vi "DllFxpSubTemp.vi"(6 "ready for output":bool, 9 "input valid":bool, 10 "y":fxp<+/-,16,1>, 11 "x":fxp<+/-,16,1>) -> (1 "output valid":bool, 2 "overflow?":bool, 3 "z":fxp<+/-,17,2> format="%.16g", 4 "ready for input":bool)   [LabVIEW 2017]
uses:
  <vilib>/rvi/FXPMathLib/FxpSub/subVIs/nifxpmath_Sub_SimConfig.ctl
  <vilib>/fxp/LVFixedPointQuantizationPolicyTypeDef.ctl
  <vilib>/fxp/LVFixedPointOverflowPolicyTypeDef.ctl
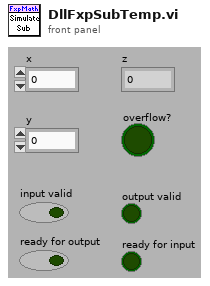
[diagram p1: front panel]
types:
  T1 = typedef "nifxpmath_Sub_SimConfig.ctl" = cluster{"kXSigned":bool, "kXWl":u32, "kXIwl":i32, "kYSigned":bool, "kYWl":u32, "kYIwl":i32, "kZSigned":bool, "kZWl":u32, "kZIwl":i32, "Fixed-Point:Quantization Policy":T2, "Fixed-Point:Overflow Policy":T3, "OutputRegister":bool, "SupportSCTL?":bool}
  T2 = typedef "LVFixedPointQuantizationPolicyTypeDef.ctl" = enum32{"Truncate", "Round-Half-Up (Asymmetric)", "Round-Half-Even"}
  T3 = typedef "LVFixedPointOverflowPolicyTypeDef.ctl" = enum32{"Wrap", "Saturate"}
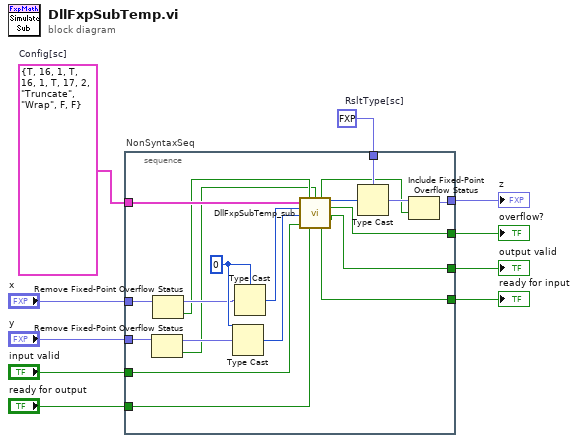
[diagram p0: block diagram]
diagram:
  w1 = T1 {"kXSigned"=TRUE, "kXWl"=16, "kXIwl"=1, "kYSigned"=TRUE, "kYWl"=16, "kYIwl"=1, "kZSigned"=TRUE, "kZWl"=17, "kZIwl"=2, "Fixed-Point:Quantization Policy"=enum."Truncate", "Fixed-Point:Overflow Policy"=enum."Wrap", "OutputRegister"=FALSE, "SupportSCTL?"=FALSE}  # Config[sc]
  w6 = fxp<+,17,2> 0.0  # RsltType[sc]
  n1 = stacked-sequence "NonSyntaxSeq" {
    tunnel: "x" -> [w19]
    tunnel: "y" -> [w16]
    tunnel: w6 -> [w30]
    tunnel: [w11] -> w5
    tunnel: "input valid" -> [w26]
    tunnel: [w24] -> w4
    tunnel: [w21] -> w2
    tunnel: [w20] -> w3
    tunnel: "ready for output" -> [w23]
    tunnel: w1 -> [w22]
    frame #0 {
      w29 = u64 0
      n2 = Remove Fixed-Point Overflow Status(3:w16) -> (0:w14:bool, 1:w15:fxp<+/-,16,1>)
      n3 = Remove Fixed-Point Overflow Status(3:w19) -> (0:w17:bool, 1:w18:fxp<+/-,16,1>)
      n4 = Type Cast(type=w29, x=w15) -> (*(type *) &x=w27:u64)
      n5 = Type Cast(type=w29, x=w18) -> (*(type *) &x=w28:u64)
      n6 = call <vilib>:"DllFxpSubTemp_sub.vi"("Config[sc]"=w22, "x ovfl status"=w17, "y ovfl status"=w14, "x"=w28, "y"=w27, "input valid"=w26, "ready for output"=w23) -> ("z ovfl status"=w12:bool, "z"=w25:u64, "operational overflow"=w24:bool, "output valid"=w20:bool, "ready for input"=w21:bool)  [unwired: 4 out]
      n7 = Type Cast(type=w30, x=w25) -> (*(type *) &x=w13:fxp<+,17,2>)
      n8 = Include Fixed-Point Overflow Status(2:w12, 3:w13) -> (1:w11:fxp<+,17,2>)
    }
  }
  "overflow?" <- w4
  "z" <- w5
  "output valid" <- w3
  "ready for input" <- w2
